vi "make uniform dot at coordinates.vi"(6 "Color":u32(colorbox)=16711680, 9 "Y":sgl, 10 "X":sgl, 11 "Refnum in":T1) -> (3 "Refnum out":T1)   [LabVIEW 2018]
uses:
  <vilib>/vision/Image Controls.llb/IMAQ Image.ctl
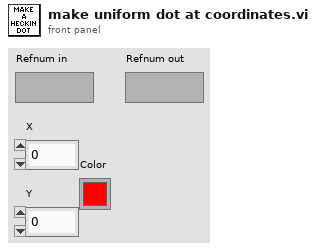
[diagram p1: front panel]
types:
  T1 = typedef "IMAQ Image.ctl" = refnum<image>
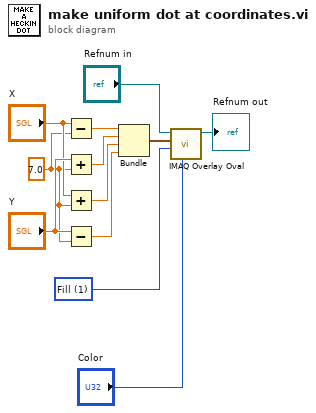
[diagram p0: block diagram]
diagram:
  w7 = u32 1 items=["Frame", "Fill"] ("Drawing Mode")
  w3 = sgl 7.0 ("y")
  n1 = Subtract(x="X", y=w3) -> (x-y=w6:sgl)
  n2 = Add(x="Y", y=w3) -> (x+y=w4:sgl)
  n3 = Add(x="X", y=w3) -> (x+y=w5:sgl)
  n4 = Subtract(x="Y", y=w3) -> (x-y=w2:sgl)
  n5 = Bundle(w6, w4, w5, w2) -> (w8:cluster{sgl, sgl, sgl, sgl})  [unwired: 1 in]
  n6 = call "IMAQ Overlay Oval"("Color"="Color", "Drawing Mode (Frame)"=w7, "Bounding Rectangle"=w8, "Image"="Refnum in") -> ("Image Out"=→"Refnum out":T1)  [unwired: 6 in, 1 out]
